vi "DAQmx Channel Name.vi"(1 "DAQmx Channel Name":refnum<k21>) -> (0 "DAQmx Task Channel Out":refnum<k21>)   [LabVIEW 2012]
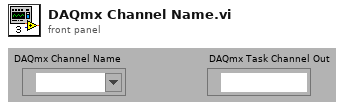
[diagram p1: front panel]
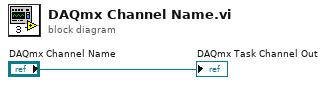
[diagram p0: block diagram]
diagram:
  "DAQmx Task Channel Out" <- "DAQmx Channel Name"
